vi "Joystick_Cluster.vi"(9 "Xbox":string="Xbox", 10 "Thrustmaster":string="Thrustmaster") -> (2 "Joystick Output":T1)   [LabVIEW 2020]
uses:
  <vilib>/Rock Robotics/WPI/Utilities/WPI_GetSetVariantRefNum.vi
panel:
  in  "Joystick Controls Cluster":T1
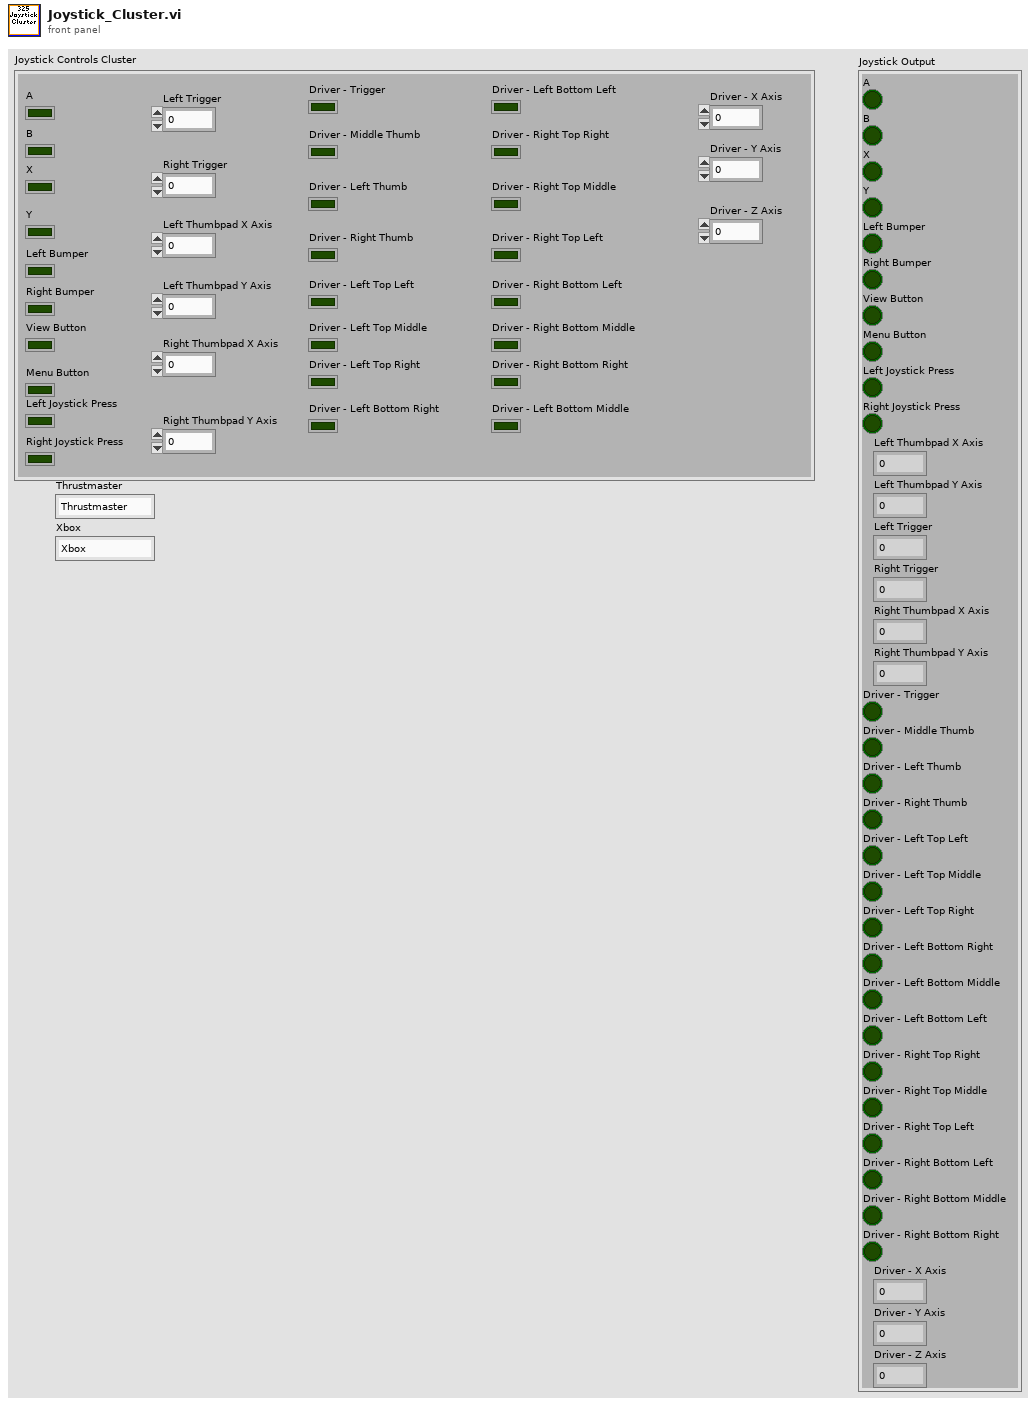
[diagram p1: front panel]
types:
  T1 = cluster{"A":bool, "B":bool, "X":bool, "Y":bool, "Left Bumper":bool, "Right Bumper":bool, "View Button":bool, "Menu Button":bool, "Left Joystick Press":bool, "Right Joystick Press":bool, "Left Thumbpad X Axis":dbl, "Left Thumbpad Y Axis":dbl, "Left Trigger":dbl, "Right Trigger":dbl, "Right Thumbpad X Axis":dbl, "Right Thumbpad Y Axis":dbl, "Driver - Trigger":bool, "Driver - Middle Thumb":bool, "Driver - Left Thumb":bool, "Driver - Right Thumb":bool, "Driver - Left Top Left ":bool, "Driver - Left Top Middle":bool, "Driver - Left Top Right":bool, "Driver - Left Bottom Right":bool, "Driver - Left Bottom Middle":bool, "Driver - Left Bottom Left":bool, "Driver - Right Top Right":bool, "Driver - Right Top Middle":bool, "Driver - Right Top Left":bool, "Driver - Right Bottom Left":bool, "Driver - Right Bottom Middle":bool, "Driver - Right Bottom Right":bool, "Driver - X Axis":dbl, "Driver - Y Axis":dbl, "Driver - Z Axis":dbl}
  T2 = typedef "WPI_JoystickDevRef.ctl" = cluster{"Device":T3}
  T3 = typedef "WPI_JoystickDeviceEnum.ctl" = enum16{"USB 0", "USB 1", "USB 2", "USB 3", "USB 4", "USB 5"}
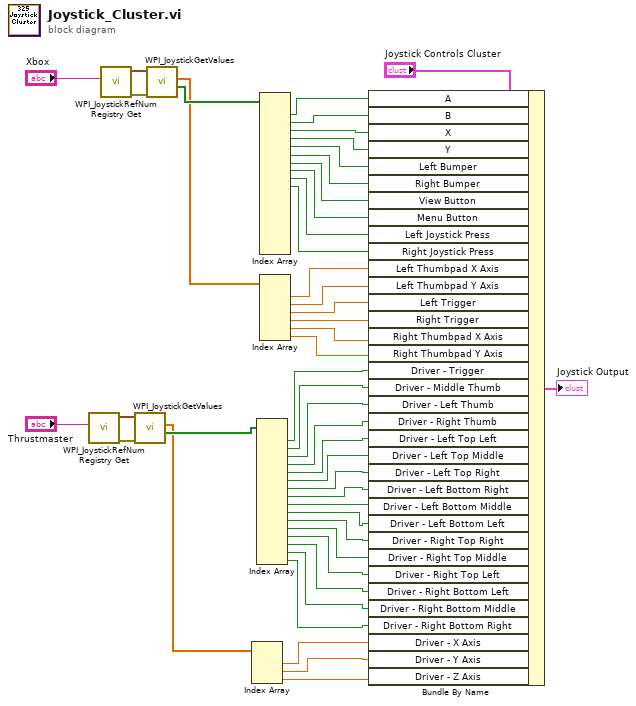
[diagram p0: block diagram]
diagram:
  n1 = call <vilib>:"WPI_JoystickRefNum Registry Get.vi"("refnum name"="Thrustmaster") -> ("error out"=w25:errorcluster, "JoystickDevRef"=w24:T2)  [unwired: 9 in]
  n2 = call <vilib>:"WPI_JoystickRefNum Registry Get.vi"("refnum name"="Xbox") -> ("error out"=w47:errorcluster, "JoystickDevRef"=w46:T2)  [unwired: 9 in]
  n3 = call <vilib>:"WPI_JoystickGetValues.vi"("error in (no error)"=w25, "JoystickDevRef"=w24) -> ("Buttons"=w22:bool[], "Axes"=w21:dbl[])  [unwired: 5 in, 3 out]
  n4 = call <vilib>:"WPI_JoystickGetValues.vi"("error in (no error)"=w47, "JoystickDevRef"=w46) -> ("Buttons"=w44:bool[], "Axes"=w32:dbl[])  [unwired: 5 in, 3 out]
  n5 = Index Array(array=w21) -> (element #1=w4:dbl, element #2=w3:dbl, element #3=w2:dbl)  [unwired: 3 in]
  n6 = Index Array(array=w22) -> (element #1=w20:bool, element #2=w19:bool, element #3=w18:bool, element #4=w17:bool, element #5=w16:bool, element #6=w15:bool, element #7=w14:bool, element #8=w13:bool, element #9=w12:bool, element #10=w11:bool, element #11=w10:bool, element #12=w9:bool, element #13=w8:bool, element #14=w7:bool, element #15=w6:bool, element #16=w5:bool)  [unwired: 16 in]
  n7 = Index Array(array=w44) -> (element #1=w43:bool, element #2=w42:bool, element #3=w41:bool, element #4=w40:bool, element #5=w38:bool, element #6=w37:bool, element #7=w36:bool, element #8=w35:bool, element #9=w34:bool, element #10=w33:bool)  [unwired: 18 in, 8 out]
  n8 = Index Array(array=w32) -> (element #1=w31:dbl, element #2=w30:dbl, element #3=w29:dbl, element #4=w28:dbl, element #5=w27:dbl, element #6=w26:dbl)  [unwired: 6 in]
  n9 = Bundle By Name(cluster="Joystick Controls Cluster", "A"=w43, "B"=w42, "X"=w41, "Y"=w40, "Left Bumper"=w38, "Right Bumper"=w37, "View Button"=w36, "Menu Button"=w35, "Left Joystick Press"=w34, "Right Joystick Press"=w33, "Left Thumbpad X Axis"=w31, "Left Thumbpad Y Axis"=w30, "Left Trigger"=w29, "Right Trigger"=w28, "Right Thumbpad X Axis"=w27, "Right Thumbpad Y Axis"=w26, "Driver - Trigger"=w20, "Driver - Middle Thumb"=w19, "Driver - Left Thumb"=w18, "Driver - Right Thumb"=w17, "Driver - Left Top Left"=w16, "Driver - Left Top Middle"=w15, "Driver - Left Top Right"=w14, "Driver - Left Bottom Right"=w13, "Driver - Left Bottom Middle"=w12, "Driver - Left Bottom Left"=w11, "Driver - Right Top Right"=w10, "Driver - Right Top Middle"=w9, "Driver - Right Top Left"=w8, "Driver - Right Bottom Left"=w7, "Driver - Right Bottom Middle"=w6, "Driver - Right Bottom Right"=w5, "Driver - X Axis"=w4, "Driver - Y Axis"=w3, "Driver - Z Axis"=w2) -> (→"Joystick Output":T1)
